vi "ExtractStats2.vi"(6 "dt":dbl, 7 "Graphs":cluster{dbl[], dbl[]}[](array[cluster]), 8 "Analytes":string[](array[string]), 10 "Bias":cluster{dbl[], dbl[]}[](array[cluster]), 11 "channel":string) -> (1 "dataTable":string[][](array[string]))   [LabVIEW 2024]
uses:
  <vilib>/Analysis/baseanly.llb/Mean (DBL).vi
  <vilib>/Analysis/NI_AALBase.lvlib
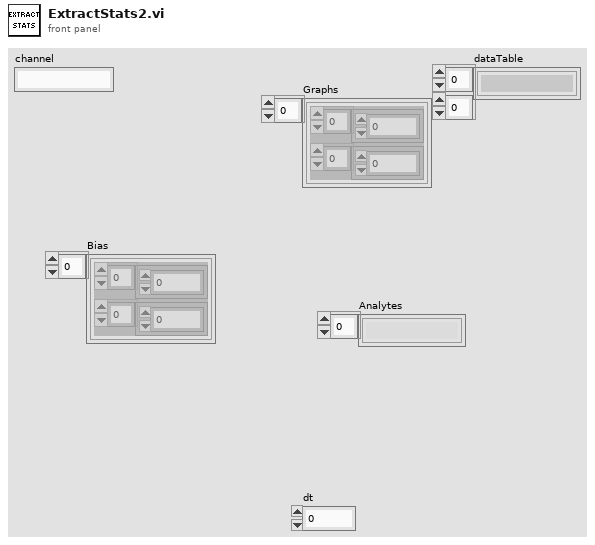
[diagram p1: front panel]
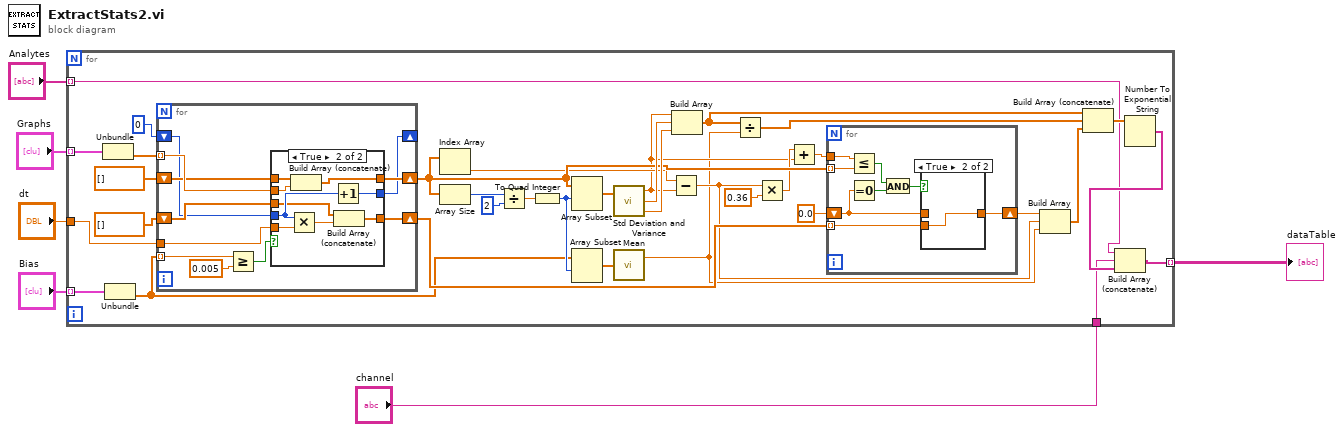
[diagram p0: block diagram]
diagram:
  n1 = for {
    tunnel: "Bias" -> [w41] mode=indexing
    tunnel: "Graphs" -> [w40] mode=indexing
    tunnel: "dt" -> [w37]
    tunnel: "Analytes" -> [w9] mode=indexing
    tunnel: "channel" -> [w8]
    tunnel: [w7] -> w1 mode=indexing
    n2 = Unbundle(w40) -> (w39:dbl[])  [unwired: 1 out]
    n3 = Unbundle(w41) -> (w11:dbl[])  [unwired: 1 out]
    n4 = for {
      tunnel: w11 -> [w52] mode=indexing
      tunnel: w39 -> [w60] mode=indexing
      shift-right: [w59] -> w24
      shift-left: dbl[] [] -> [w58]
      shift-right: [w57] -> w23
      shift-left: dbl[] [] -> [w56]
      tunnel: w37 -> [w53]
      shift-right: [w54] -> _
      shift-left: 0 -> [w55]
      n5 = Greater Or Equal?(x=w52, y=0.005) -> (x >= y?=w61:bool)
      n6 = case shown="True" w61 {
        tunnel: w60 -> [_ w66]
        tunnel: [w65 w74] -> w59
        tunnel: w58 -> [w65 w73]
        tunnel: [w64 w68] -> w57
        tunnel: w56 -> [w64 w67]
        tunnel: w55 -> [w63 w71]
        tunnel: [w63 w72] -> w54
        tunnel: w53 -> [_ w70]
        frame False {
        }
        frame True {
          n7 = Multiply(x=w71, y=w70) -> (x*y=w69:dbl)
          n8 = Build Array (concatenate)(w73, w66) -> (w74:dbl[])
          n9 = Increment(x=w71) -> (x+1=w72:i32)
          n10 = Build Array (concatenate)(w67, w69) -> (w68:dbl[])
        }
      }
    }
    n11 = Index Array(array=w24) -> (element=w21:dbl)  [unwired: 1 in]
    n12 = Array Size(array=w24) -> (size(s)=w34:i32)
    n13 = Divide(x=w34, y=2) -> (x/y=w32:dbl)
    n14 = To Quad Integer(1:w32) -> (0:w31:i64)
    n15 = Array Subset(array=w24, index=w31) -> (w29:dbl[])  [unwired: 1 in]
    n16 = Array Subset(array=w11, index=w31) -> (w30:dbl[])  [unwired: 1 in]
    n17 = call <vilib>:"Std Deviation and Variance.vi"("X"=w29) -> ("mean"=w14:dbl, "standard deviation"=w28:dbl, "variance"=w27:dbl)  [unwired: 1 in]
    n18 = call-poly <vilib>:"Mean.vi"("X"=w30) -> ("mean"=w13:dbl)  [unwired: 1 out]
    n19 = Subtract(x=w21, y=w14) -> (x-y=w16:dbl)
    n20 = Build Array(w14, w28, w27) -> (w26:dbl[])
    n21 = Divide(x=w26, y=w13) -> (x/y=w25:dbl[])
    n22 = Multiply(x=w16, y=0.36) -> (x*y=w19:dbl)
    n23 = Add(x=w19, y=w14) -> (x+y=w18:dbl)
    n24 = for {
      tunnel: w24 -> [w48] mode=indexing
      tunnel: w23 -> [w42] mode=indexing
      tunnel: w18 -> [w49]
      shift-right: [w46] -> w17
      shift-left: 0.0 -> [w44]
      n25 = Less Or Equal?(x=w49, y=w48) -> (x <= y?=w47:bool)
      n26 = Equal To 0?(x=w44) -> (x = 0?=w43:bool)
      n27 = And(x=w47, y=w43) -> (x .and. y?=w45:bool)
      n28 = case shown="True" w45 {
        tunnel: [w50 w51] -> w46
        tunnel: w44 -> [w50 _]
        tunnel: w42 -> [_ w51]
        frame False {
        }
        frame True {
        }
      }
    }
    n29 = Build Array(w17, w16, w13) -> (w15:dbl[])
    n30 = Build Array (concatenate)(w26, w25, w15) -> (w12:dbl[])
    n31 = Number To Exponential String(number=w12) -> (E-format string=w10:string[])  [unwired: 3 in]
    n32 = Build Array (concatenate)(w9, w8, w10) -> (w7:string[])
  }
  "dataTable" <- w1
